vi "variavelVelocidades.vi"() -> ()   [LabVIEW 2023]
panel:
  in  "velocidadeMaxima":dbl
  in  "velocidadePadrao":dbl
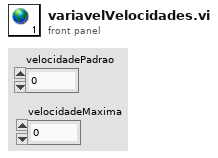
[diagram p1: front panel]
diagram:
